vi "InsertIntoNewProperty.vi"(5 "$Path or Item Name":string, 6 "JSON Items":string[](array[string]), 7 "JSON In":string, 8 "error in (no error)":errorcluster, 9 "Item Names":string[](array[string]), 10 "index":i32, 11 "Input array":string[](array[string])) -> (0 "error out":errorcluster, 3 "<JSON>":string)   [LabVIEW 2017]
uses:
  <vilib>/JDP Science/JSONtext/JSONtext.lvlib
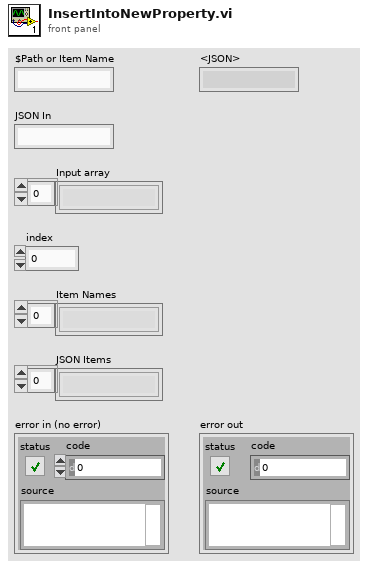
[diagram p1: front panel]
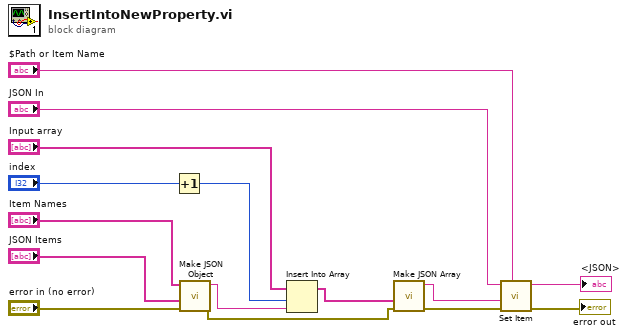
[diagram p0: block diagram]
diagram:
  n1 = Increment(x="index") -> (x+1=w1:i32)
  n2 = call <vilib>:"Make JSON Object.vi"("error in (no error)"="error in (no error)", "JSON Items"="JSON Items", "Item Names"="Item Names") -> ("error out"=w7:errorcluster, "<JSON>"=w3:string)  [unwired: 7 in]
  n3 = Insert Into Array(array="Input array", index=w1, new element=w3) -> (w6:string[])
  n4 = call <vilib>:"Make JSON Array.vi"("error in (no error)"=w7, "JSON Elements"=w6) -> ("error out"=w9:errorcluster, "<JSON>"=w8:string)  [unwired: 8 in]
  n5 = call <vilib>:"Set Item.vi"("$Path or Item Name"="$Path or Item Name", "error in (no error)"=w9, "JSON to Insert"=w8, "JSON"="JSON In") -> ("error out"=→"error out":errorcluster, "<JSON>"=→"<JSON>":string)  [unwired: 4 in, 1 out]
